vi "String_to_date.vi"(1 "String":string[](array[string])) -> (0 "Date":timestamp[](array[timestamp]))   [LabVIEW 2024]
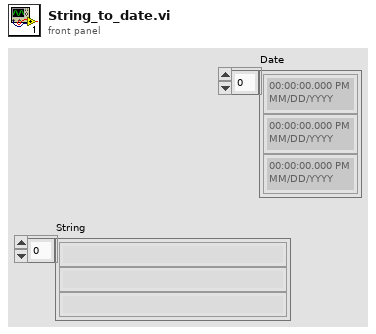
[diagram p1: front panel]
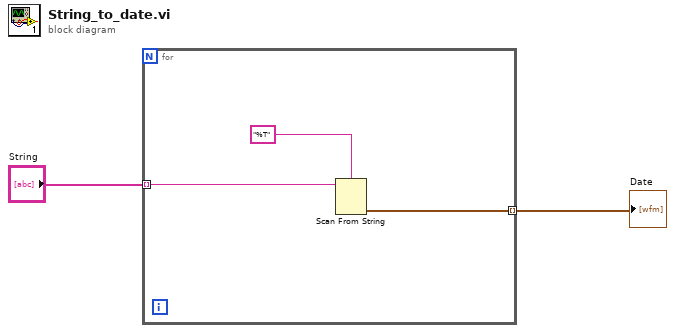
[diagram p0: block diagram]
diagram:
  n1 = for {
    tunnel: "String" -> [w4] mode=indexing
    tunnel: [w3] -> w1 mode=indexing
    n2 = Scan From String(format string="%T", input string=w4) -> (output 1=w3:timestamp)  [unwired: 3 in, 3 out]
  }
  "Date" <- w1
